vi "Check Message Pending.vi"(11 "Data Array":u8[](array[numeric])) -> (3 "x .and. y?":bool)   [LabVIEW 2018]
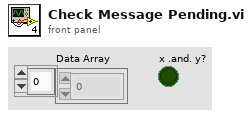
[diagram p1: front panel]
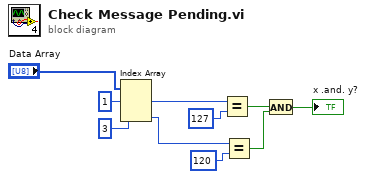
[diagram p0: block diagram]
diagram:
  n1 = Index Array(array="Data Array", index #1=1 ("index"), index #3=3 ("index")) -> (element #1=w3:u8, element #3=w7:u8)  [unwired: 1 in, 1 out]
  n2 = Equal?(x=w3, y=u8 127 ("Numeric")) -> (x = y?=w8:bool)
  n3 = Equal?(x=w7, y=u8 120 ("Numeric")) -> (x = y?=w9:bool)
  n4 = And(x=w8, y=w9) -> (x .and. y?=→"x .and. y?":bool)
